vi "Register Service.vi"(8 "error in (no error)":errorcluster, 10 "Service":refnum<class "Service.lvclass">, 11 "Vecto in":refnum<class "Vecto.lvclass">) -> (0 "error out":errorcluster, 3 "Vecto out":refnum<class "Vecto.lvclass">)   [LabVIEW 2020, in "Vecto.lvlib" / "Vecto.lvclass"]
uses:
  Vecto.lvclass
  Service/Service.lvclass
  <vilib>/IlluminatedG/IG HTTP Server/HTTP Server/Service/Service.lvclass
  Vecto.lvclass/Vecto.ctl
  Service Container/Service Container.lvclass
  <vilib>/IlluminatedG/IG HTTP Server/HTTP Server/Server/Server.lvclass
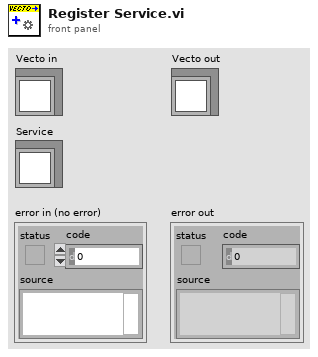
[diagram p1: front panel]
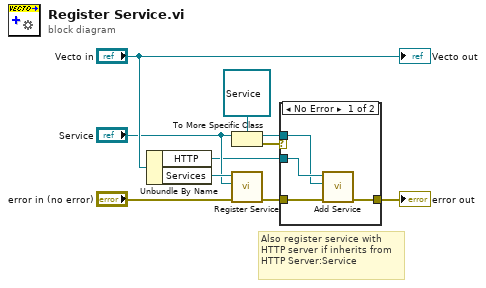
[diagram p0: block diagram]
diagram:
  # "Also register service with HTTP server if inherits from HTTP Server:Service"
  n1 = Unbundle By Name("Vecto in") -> ("HTTP"=w2:refnum<class "Server.lvclass">, "Services"=w9:refnum<class "Service Container.lvclass">)
  n2 = To More Specific Class(target class=refnum<class "Service.lvclass"> refnum ("HTTP Server:Service.lvclass"), reference="Service") -> (specific class reference=w4:refnum<class "Service.lvclass">, error out=w5:errorcluster)  [unwired: 1 in]
  n3 = call "Register Service.vi"("error in (no error)"="error in (no error)", "Service"="Service", "Service Container in"=w9) -> ("error out"=w6:errorcluster)  [unwired: 7 in, 1 out]
  n4 = case shown="No Error" w5 {
    tunnel: w6 -> [w14 w15]
    tunnel: w4 -> [w12 _]
    tunnel: w2 -> [w13 _]
    tunnel: [w11 w15] -> w1
    frame No Error {
      n5 = call <vilib>:"Add Service.vi"("error in (no error)"=w14, "Service"=w12, "Server in"=w13) -> ("error out"=w11:errorcluster)  [unwired: 7 in, 1 out]
    }
    frame Error {
    }
  }
  "error out" <- w1
  "Vecto out" <- "Vecto in"
